vi "ArduinoBox_handle_ae.vi"(10 "VISA resource In":refnum<visa-resource-name>, 11 "Enum":enum16{"WRITE", "READ"}(ring)) -> (3 "VISA resource Out":refnum<visa-resource-name>)   [LabVIEW 2014]
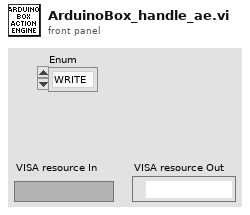
[diagram p1: front panel]
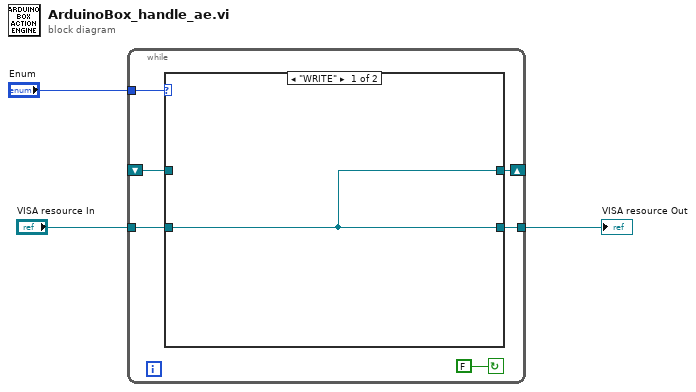
[diagram p0: block diagram]
diagram:
  n1 = while {
    tunnel: "Enum" -> [w8]
    shift-right: [w4] -> _
    shift-left: _ -> [w7]
    tunnel: "VISA resource In" -> [w6]
    tunnel: [w5] -> w2
    stop <- FALSE continue-if-true
    n2 = case shown="\"WRITE\"" w8 {
      tunnel: w7 -> [_ w11]
      tunnel: w6 -> [w10 _]
      tunnel: [w10 w11] -> w5
      tunnel: [w10 w11] -> w4
      frame "WRITE" {
      }
      frame "READ" {
      }
    }
  }
  "VISA resource Out" <- w2
